vi "Code Contains Secrets--error.vi"(4 "error in":errorcluster) -> (0 "error out":errorcluster)   [LabVIEW 2025]
doc: "Custom error -8000: the analyzed code contains one or more secrets."
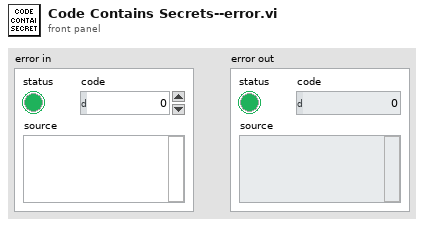
[diagram p1: front panel]
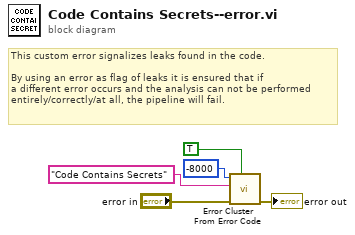
[diagram p0: block diagram]
diagram:
  # "This custom error signalizes leaks found in the code.\n\nBy using an error as flag of leaks it is ensured that if\na different error occurs and the analysis can not be performed\nentirely/correctly/at all, the pipeline will fail."
  n1 = call <vilib>:"Error Cluster From Error Code.vi"("show call chain? (False)"=TRUE, "error in (no error)"="error in", "error message (\"\")"="Code Contains Secrets" ("format string"), "error code (0)"=-8000) -> ("error out"=→"error out":errorcluster)  [unwired: 5 in]
